vi "身份证识别.vi"() -> ()   [LabVIEW 2018]
uses:
  <vilib>/userdefined/High Color/IMAQdx.ctl
  <vilib>/vision/NI_Vision_Development_Module.lvlib
  <vilib>/vision/driver/NI_Vision_Acquisition_Software.lvlib
panel:
  out "公民身份号码":string
  out "住址":string
  out "出生":string
  out "民族":string
  out "性别":string
  out "姓名":string
  in  "读卡":bool
  out "Image":T1(plugin-control)
  in  "摄像头":bool
  in  "打开":bool
  in  "训练":bool
  in  "修正成为":string
  in  "停止按钮":bool
  out "Read String":string
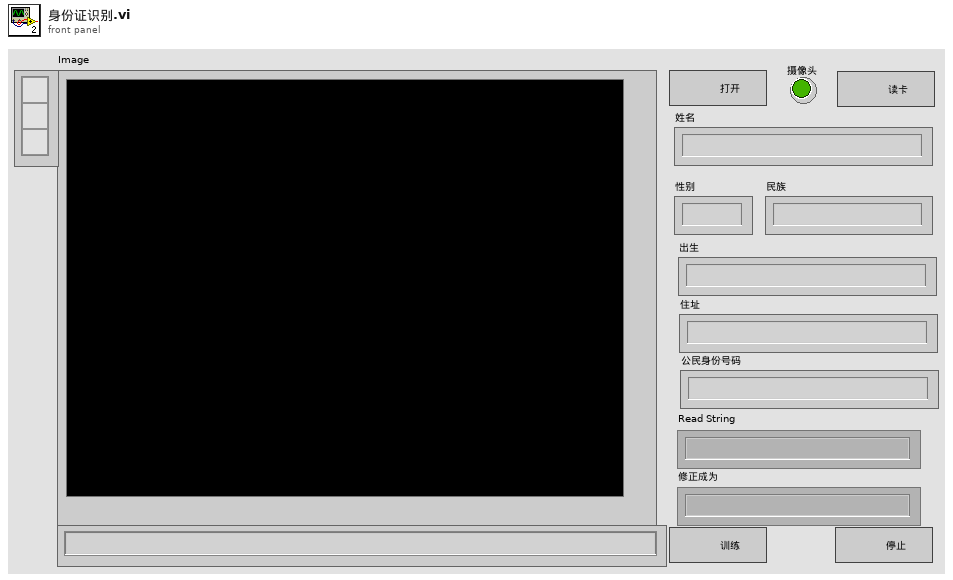
[diagram p1: front panel]
types:
  T1 = typedef "IMAQ Image.ctl" = refnum<image>
  T2 = cluster{"Global Rectangle":i32[], "Contours":cluster{"Contour Type":u32, "ROI Type":u32, "Points":i32[]}[]}
  T3 = typedef "IMAQdx.ctl" = refnum<k21>
  T4 = typedef "Image Type" = u32
  T5 = typedef "IMAQ OCR Session.ctl" = refnum<k1>
  T6 = cluster{"Global Rectangle":i32[], "Contours":cluster{"Contour Type":u32, "ROI Type":u32, "Points":i32[]}[]}[]
  T7 = cluster{"Left":i32, "Top":i32, "Right":i32, "Bottom":i32}
  T8 = cluster{"Global Rectangle":i32[], "Contours":cluster{"ID":enum32{"External", "Internal"}, "Type":u32, "Coordinates":i32[]}[]}
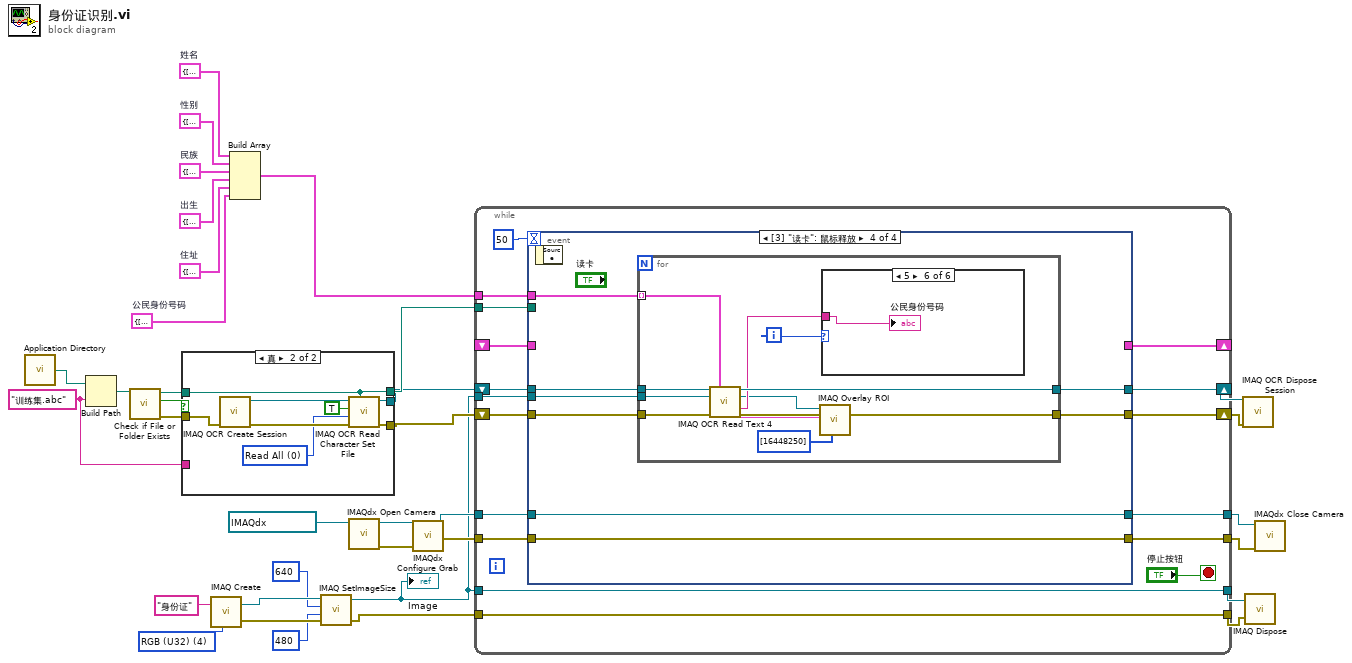
[diagram p0: block diagram]
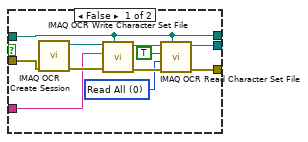
[diagram p2: hidden frame]
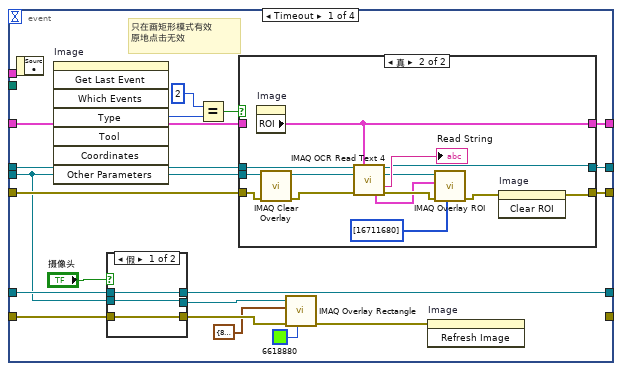
[diagram p3: hidden frame]
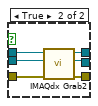
[diagram p4: hidden frame]
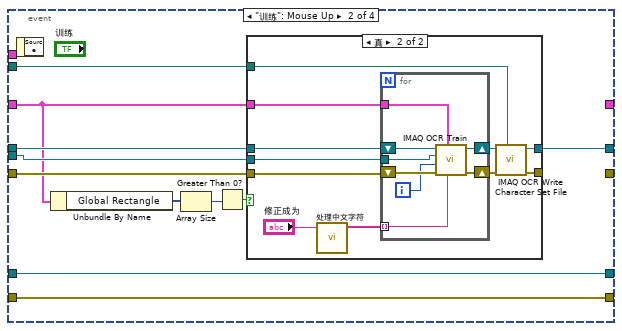
[diagram p6: hidden frame]
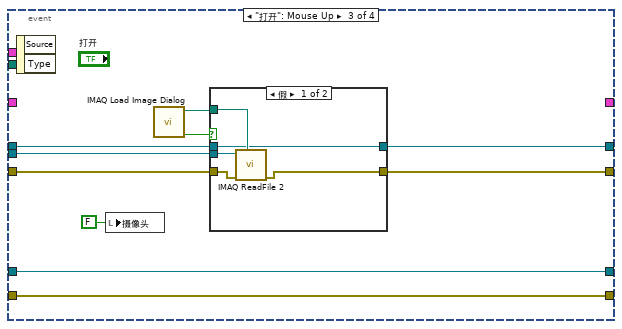
[diagram p8: hidden frame]
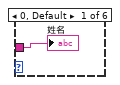
[diagram p10: hidden frame]
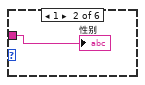
[diagram p11: hidden frame]
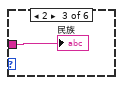
[diagram p12: hidden frame]
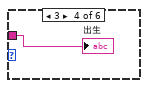
[diagram p13: hidden frame]
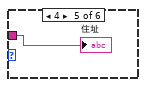
[diagram p14: hidden frame]
diagram:
  w1 = T2 {"Global Rectangle"=[198, 361, 601, 411], "Contours"=[{"Contour Type"=0, "ROI Type"=3, "Points"=[198, 361, 601, 411]}]}  # 公民身份号码
  w2 = T2 {"Global Rectangle"=[119, 243, 382, 359], "Contours"=[{"Contour Type"=0, "ROI Type"=3, "Points"=[119, 243, 382, 359]}]}  # 住址
  w3 = T2 {"Global Rectangle"=[111, 189, 381, 225], "Contours"=[{"Contour Type"=0, "ROI Type"=3, "Points"=[111, 189, 381, 225]}]}  # 出生
  w4 = T2 {"Global Rectangle"=[245, 144, 404, 180], "Contours"=[{"Contour Type"=0, "ROI Type"=3, "Points"=[245, 144, 404, 180]}]}  # 民族
  w5 = T2 {"Global Rectangle"=[109, 142, 189, 181], "Contours"=[{"Contour Type"=0, "ROI Type"=3, "Points"=[109, 142, 189, 181]}]}  # 性别
  w6 = T2 {"Global Rectangle"=[118, 79, 398, 137], "Contours"=[{"Contour Type"=0, "ROI Type"=3, "Points"=[118, 79, 398, 137]}]}  # 姓名
  w24 = "训练集.abc" ("名称或相对路径")
  w30 = T4 4 items=["Grayscale (U8)", "Grayscale (I16)", "Grayscale (SGL)", "Complex (CSG)", "RGB (U32)", "HSL (U32)", "RGB (U64)", "Grayscale (U16)"] ("Image Type")
  n1 = call <vilib>:"Application Directory.vi"() -> ("Application Directory"=w29:path)
  n2 = Build Path(base path=w29, name or relative path=w24) -> (appended path=w28:path)
  n3 = call <vilib>:"Check if File or Folder Exists.vi"("path"=w28) -> ("error out"=w25:errorcluster, "file or folder exists?"=w26:bool, "dup path"=w27:path)  [unwired: 8 in]
  n4 = case shown="真" w26 {
    tunnel: w27 -> [w36 w47]
    tunnel: w25 -> [w43 w50]
    tunnel: w24 -> [w44 _]
    tunnel: [w42 w52] -> w22
    tunnel: [w41 w51] -> w21
    tunnel: [w36 w47] -> w23
    frame False {
      w37 = 0 items=["Read All", "Read Character Set Only", "Read Properties Only"] ("Read Options")
      n5 = call "IMAQ OCR Create Session"("error in (no error)"=w43) -> ("error out"=w46:errorcluster, "IMAQ OCR Session"=w45:T5)  [unwired: 9 in]
      n6 = call "IMAQ OCR Write Character Set File"("File Path"=w36, "error in (no error)"=w46, "Character Set Description"=w44, "IMAQ OCR Session"=w45) -> ("error out"=w39:errorcluster, "IMAQ OCR Session (dup)"=w40:T5)  [unwired: 6 in]
      n7 = call "IMAQ OCR Read Character Set File"("File Path"=w36, "error in (no error)"=w39, "Read Options"=w37, "Append To Character Set? (F)"=TRUE, "IMAQ OCR Session"=w40) -> ("error out"=w41:errorcluster, "IMAQ OCR Session (dup)"=w42:T5)  [unwired: 4 in, 1 out]
    }
    frame True {
      w48 = 0 items=["Read All", "Read Character Set Only", "Read Properties Only"] ("Read Options")
      n8 = call "IMAQ OCR Create Session"("error in (no error)"=w50) -> ("error out"=w54:errorcluster, "IMAQ OCR Session"=w53:T5)  [unwired: 9 in]
      n9 = call "IMAQ OCR Read Character Set File"("File Path"=w47, "error in (no error)"=w54, "Read Options"=w48, "Append To Character Set? (F)"=TRUE, "IMAQ OCR Session"=w53) -> ("error out"=w51:errorcluster, "IMAQ OCR Session (dup)"=w52:T5)  [unwired: 4 in, 1 out]
    }
  }
  n10 = call "IMAQ Create"("Image Name"="身份证", "Image Type"=w30) -> ("New Image"=w13:T1, "error out"=w12:errorcluster)  [unwired: 3 in]
  n11 = Build Array(w6, w5, w4, w3, w2, w1) -> (w7:T6)
  n12 = call "IMAQ SetImageSize"("error in (no error)"=w12, "Y Resolution"=480, "X Resolution"=640, "Image"=w13) -> ("error out"=w9:errorcluster, "Image Out"=w8:T1)  [unwired: 1 in]
  "Image" <- w8
  n13 = call <vilib>:"IMAQdx Open Camera.vi"("Session In"=T3 "手机摄像头") -> ("error out"=w18:errorcluster, "Session Out"=w19:T3)  [unwired: 9 in]
  n14 = call <vilib>:"IMAQdx Configure Grab.vi"("error in"=w18, "Session In"=w19) -> ("error out"=w16:errorcluster, "Session Out"=w17:T3)  [unwired: 8 in]
  n15 = while {
    tunnel: w8 -> [w67]
    shift-right: [w69] -> w35
    shift-left: w22 -> [w71]
    shift-right: [w68] -> w34
    shift-left: w21 -> [w70]
    tunnel: w9 -> [w56]
    tunnel: w8 -> [w57]
    tunnel: [w57] -> w32
    tunnel: [w56] -> w31
    tunnel: w23 -> [w65]
    shift-right: [w63] -> _
    shift-left: _ -> [w62]
    tunnel: w17 -> [w61]
    tunnel: w16 -> [w60]
    tunnel: [w59] -> w14
    tunnel: [w58] -> w15
    tunnel: w7 -> [w55]
    stop <- "停止按钮" stop-if-true
    n16 = event shown="[3] \"读卡\": 鼠标释放" {
      selector: _ -> [_ _ _ _]
      dyn-events: _ -> [_ _ _ _]
      timeout: 50 -> [_ _ _ _]
      tunnel: w71 -> [w90 w127 w156 w173]
      tunnel: w70 -> [w89 w125 w157 w172]
      tunnel: [w88 w126 w155 w169] -> w69
      tunnel: [w87 _ w154 w168] -> w68
      tunnel: w67 -> [w80 w124 w158 w171]
      tunnel: w65 -> [_ w119 _ _]
      tunnel: [w85 _ _ _] -> w63
      tunnel: w62 -> [w83 w123 _ _]
      tunnel: w61 -> [w82 w118 w153 w167]
      tunnel: w60 -> [w81 w117 w152 w166]
      tunnel: [w76 w118 w153 w167] -> w59
      tunnel: [_ w117 w152 w166] -> w58
      tunnel: w55 -> [_ _ _ w170]
      event Timeout {
        # "只在画矩形模式有效\n原地点击无效"
        n17 = event-data() -> ()  [unwired: 1 in, 1 out]
        n18 = invoke on="Image" class="ImageControl" method="Get Last Event"() -> ("Type"=w78:i32)  [unwired: 8 in, 7 out]
        n19 = case shown="假" "摄像头" {
          tunnel: w82 -> [w93 w99]
          tunnel: w81 -> [w92 w98]
          tunnel: w80 -> [w91 w97]
          tunnel: [w93 w96] -> w76
          tunnel: [w92 w95] -> w75
          tunnel: [w91 w94] -> w74
          frame False {
          }
          frame True {
            n20 = call <vilib>:"IMAQdx Grab2.vi"("error in"=w98, "Image In"=w97, "Session In"=w99) -> ("error out"=w95:errorcluster, "Image Out"=w94:T1, "Session Out"=w96:T3)  [unwired: 5 in, 1 out]
          }
        }
        n21 = Equal?(x=2, y=w78) -> (x = y?=w86:bool)
        n22 = case shown="真" w86 {
          tunnel: w90 -> [w102 w116]
          tunnel: w89 -> [w100 w110]
          tunnel: [w102 w106] -> w88
          tunnel: [w100 w103] -> w87
          tunnel: w80 -> [_ w112]
          tunnel: [w101 w105] -> w85
          tunnel: w83 -> [w101 _]
          frame False {
          }
          frame True {
            n23 = property on="Image" class="ImageControl"() -> ("ROI"=w105:T2)  [unwired: 2 in, 2 out]
            n24 = call "IMAQ Clear Overlay"("error in (no error)"=w110, "Image"=w112) -> ("error out"=w109:errorcluster, "Image Out"=w111:T1)  [unwired: 8 in]
            n25 = call "IMAQ OCR Read Text 4"("IMAQ OCR Session"=w116, "ROI Descriptor"=w105, "Image"=w111, "error in (no error)"=w109) -> ("IMAQ OCR Session (dup)"=w106:T5, "Image (dup)"=w114:T1, "Read String"=→"Read String":string, "ROI Bounding Characters"=w107:T8, "error out"=w108:errorcluster)  [unwired: 5 in, 2 out]
            n26 = call "IMAQ Overlay ROI"("Colors (Green)"=u32[] [16711680], "error in (no error)"=w108, "ROI Descriptor"=w107, "Image"=w114) -> ("error out"=w104:errorcluster)  [unwired: 6 in, 1 out]
            n27 = invoke on="Image" class="ImageControl" method="Clear ROI"(error in=w104) -> (error out=w103:errorcluster)  [unwired: 2 in, 2 out]
          }
        }
        n28 = call "IMAQ Overlay Rectangle"("Color"=u32 6618880, "error in (no error)"=w75, "Rectangle"=T7 {"Left"=8, "Top"=43, "Right"=632, "Bottom"=436}, "Image"=w74) -> ("error out"=w73:errorcluster)  [unwired: 6 in, 1 out]
        n29 = invoke on="Image" class="ImageControl" method="Refresh Image"(error in=w73) -> ()  [unwired: 2 in, 3 out]
      }
      event "训练": Mouse Up {
        n30 = event-data() -> ()  [unwired: 1 in, 1 out]
        n31 = Unbundle By Name(w123) -> ("Global Rectangle"=w122:i32[])
        n32 = Array Size(array=w122) -> (size(s)=w121:i32)
        n33 = Greater Than 0?(x=w121) -> (x > 0?=w120:bool)
        n34 = case shown="真" w120 {
          tunnel: w127 -> [w129 w138]
          tunnel: [w129 w137] -> w126
          tunnel: [w128 w136] -> _
          tunnel: w125 -> [w128 w135]
          tunnel: w124 -> [_ w134]
          tunnel: w123 -> [_ w133]
          tunnel: w119 -> [_ w132]
          frame False {
          }
          frame True {
            n35 = call "处理中文字符.vi"("字符"="修正成为") -> ("标签"=w130:string[])  [unwired: 10 in]
            n36 = for {
              shift-right: [w147] -> w139
              shift-left: w138 -> [w148]
              shift-right: [w144] -> w140
              shift-left: w135 -> [w146]
              tunnel: w134 -> [w143]
              tunnel: w133 -> [w142]
              tunnel: w130 -> [w141] mode=indexing
              i -> [w145]
              n37 = call "IMAQ OCR Train"("Character Value"=w141, "ROI Descriptor"=w142, "error in (no error)"=w146, "Object Index"=w145, "Image"=w143, "IMAQ OCR Session"=w148) -> ("error out"=w144:errorcluster, "IMAQ OCR Session (dup)"=w147:T5)  [unwired: 3 in, 1 out]
            }
            n38 = call "IMAQ OCR Write Character Set File"("File Path"=w132, "error in (no error)"=w140, "IMAQ OCR Session"=w139) -> ("error out"=w136:errorcluster, "IMAQ OCR Session (dup)"=w137:T5)  [unwired: 7 in]
          }
        }
      }
      event "打开": Mouse Up {
        n39 = event-data() -> ()  [unwired: 1 in, 2 out]
        n40 = local write "摄像头"(FALSE ("摄像头")) -> ()
        n41 = call "IMAQ Load Image Dialog"() -> ("Cancelled?"=w150:bool, "Path"=w151:path)  [unwired: 9 in, 1 out]
        n42 = case shown="假" w150 {
          tunnel: w151 -> [w163 _]
          tunnel: w158 -> [w162 _]
          tunnel: w157 -> [w161 w164]
          tunnel: w156 -> [w160 w165]
          tunnel: [w160 w165] -> w155
          tunnel: [w159 w164] -> w154
          frame False {
            n43 = call "IMAQ ReadFile 2"("File Path"=w163, "error in (no error)"=w161, "Image"=w162) -> ("error out"=w159:errorcluster)  [unwired: 4 in, 4 out]
          }
          frame True {
          }
        }
      }
      event "读卡": Mouse Up {
        n44 = event-data() -> ()  [unwired: 1 in, 1 out]
        n45 = for {
          tunnel: w173 -> [w184]
          tunnel: w172 -> [w183]
          tunnel: w171 -> [w181]
          tunnel: w170 -> [w182] mode=indexing
          tunnel: [w179] -> w169
          tunnel: [w178] -> w168
          i -> [w180]
          n46 = call "IMAQ OCR Read Text 4"("IMAQ OCR Session"=w184, "ROI Descriptor"=w182, "Image"=w181, "error in (no error)"=w183) -> ("IMAQ OCR Session (dup)"=w179:T5, "Image (dup)"=w176:T1, "Read String"=w177:string, "ROI Bounding Characters"=w175:T8, "error out"=w178:errorcluster)  [unwired: 5 in, 2 out]
          n47 = call "IMAQ Overlay ROI"("Colors (Green)"=u32[] [16448250], "ROI Descriptor"=w175, "Image"=w176) -> ()  [unwired: 7 in, 2 out]
          n48 = case shown="5" w180 {
            tunnel: w177 -> [w185 w186 w187 w188 w189 w190]
            frame 0, Default {
              "姓名" <- w185
            }
            frame 1 {
              "性别" <- w186
            }
            frame 2 {
              "民族" <- w187
            }
            frame 3 {
              "出生" <- w188
            }
            frame 4 {
              "住址" <- w189
            }
            frame 5 {
              "公民身份号码" <- w190
            }
          }
        }
      }
    }
  }
  n49 = call "IMAQ OCR Dispose Session"("error in (no error)"=w34, "IMAQ OCR Session"=w35) -> ()  [unwired: 9 in, 1 out]
  n50 = call "IMAQ Dispose"("Image"=w32, "error in (no error)"=w31) -> ()  [unwired: 4 in, 1 out]
  n51 = call <vilib>:"IMAQdx Close Camera.vi"("error in"=w15, "Session In"=w14) -> ()  [unwired: 9 in, 1 out]
